vi "Periodic Tasks.vi"   [LabVIEW 2012]
doc: "This VI runs in parallel to other tasks. It can contain as many user-defined periodic loops as you need. These can carry out PID or other sorts of timed response."
uses:
  <vilib>/Rock Robotics/SystemInterfaces/Utilities/FPGA_UtilitiesLED Source.ctl
  <vilib>/Rock Robotics/SystemInterfaces/Utilities/FPGA_UtilitiesLED State.ctl
  Robot Global Data.vi
types:
  T1 = cluster{"Case":dbl, "VisionTrack":bool, "ShootEnableWheels":bool, "Shoot":bool, "ManualExtend":dbl, "ManualRotate":dbl, "YCoord":dbl, "FlipUp":bool, "RotDeadband":dbl, "ExtDeadband":dbl, "ExtPOT":dbl, "RotPOT":dbl, "WheelFSpd":dbl, "WheelBSpd":dbl, "ServoPositions":cluster{"FlipperLeftUp":dbl, "FlipperLeftDown":dbl, "FlipperRightUp":dbl, "FlipperRightDown":dbl, "KickerLeftBack":dbl, "KickerLeftForward":dbl, "KickerRightBack":dbl, "KickerRightForward":dbl}, "POTPositions":cluster{"Setpoint 1":dbl, "Setpoint 2":dbl, "Setpoint 3":dbl, "Setpoint 4":dbl, "RotLow":dbl, "RotHigh":dbl, "ExtLow":dbl, "ExtHigh":dbl}, "ClimberHooked":bool}
  T2 = typedef "WPI_DigitalInputDevRef.ctl" = cluster{"DevStatus":errorcluster, "DIO Channel":T3, "Digital Module":T4}
  T3 = typedef "FPGA_DIOChannel.ctl" = enum8{"DIO 1", "DIO 2", "DIO 3", "DIO 4", "DIO 5", "DIO 6", "DIO 7", "DIO 8", "DIO 9", "DIO 10", "DIO 11", "DIO 12", "DIO 13", "DIO 14", "Invalid"}
  T4 = typedef "FPGA_TypedefDigitalModule.ctl" = enum16{"Digital Module 1", "Digital Module 2"}
  T5 = cluster{"FlipperLeftUp":dbl, "FlipperLeftDown":dbl, "FlipperRightUp":dbl, "FlipperRightDown":dbl, "KickerLeftBack":dbl, "KickerLeftForward":dbl, "KickerRightBack":dbl, "KickerRightForward":dbl}
  T6 = cluster{"Setpoint 1":dbl, "Setpoint 2":dbl, "Setpoint 3":dbl, "Setpoint 4":dbl, "RotLow":dbl, "RotHigh":dbl, "ExtLow":dbl, "ExtHigh":dbl}
  T7 = typedef "WPI_AnalogChannelDevRef.ctl" = cluster{"DevStatus":errorcluster, "Analog Module":T8, "Analog Channel":T9}
  T8 = typedef "FPGA_TypedefAnalogModule.ctl" = enum16{"Analog Module 1", "Analog Module 2"}
  T9 = typedef "FPGA_AIChannel.ctl" = enum8{"AI 1", "AI 2", "AI 3", "AI 4", "AI 5", "AI 6", "AI 7", "AI 8", "Invalid"}
  T10 = typedef "WPI_RelayValue.ctl" = enum16{"Off", "On", "Forward", "Reverse"}
  T11 = cluster{"Case":dbl, "Extension":dbl, "Rotation":dbl, "WheelF":dbl, "WheelB":dbl, "Left Kicker":dbl, "Right Kicker":dbl, "Left Flipper":dbl, "Right Flipper":dbl, "Lights":T10}
  T12 = typedef "WPI_GyroDevRef.ctl" = cluster{"DevStatus":errorcluster, "Analog Module":T8, "Analog Channel":T9, "Offset":dbl, "Gain (VoltsPerDegree/Second)":dbl}
  T13 = typedef "WPI_EncoderDevRef.ctl" = cluster{"DevStatus":errorcluster, "EncoderIndex":T14, "CounterIndex":T15, "DistancePerCount":dbl, "Decoding Type":T16}
  T14 = typedef "FPGA_EncoderIdx.ctl" = enum8{"Enc 0", "Enc 1", "Enc 2", "Enc 3", "Invalid"}
  T15 = typedef "FPGA_CounterCtrSystemIndex.ctl" = enum8{"Ctr 0", "Ctr 1", "Ctr 2", "Ctr 3", "Ctr 4", "Ctr 5", "Ctr 6", "Ctr 7", "Invalid"}
  T16 = typedef "WPI_EncoderType.ctl" = enum16{"1x", "2x", "4x"}
  T17 = typedef "FPGA_UtilitiesLED State.ctl" = enum16{"Off", "On", "Toggle"}
  T18 = typedef "FPGA_UtilitiesLED Source.ctl" = enum16{"User LED", "FPGA LED"}
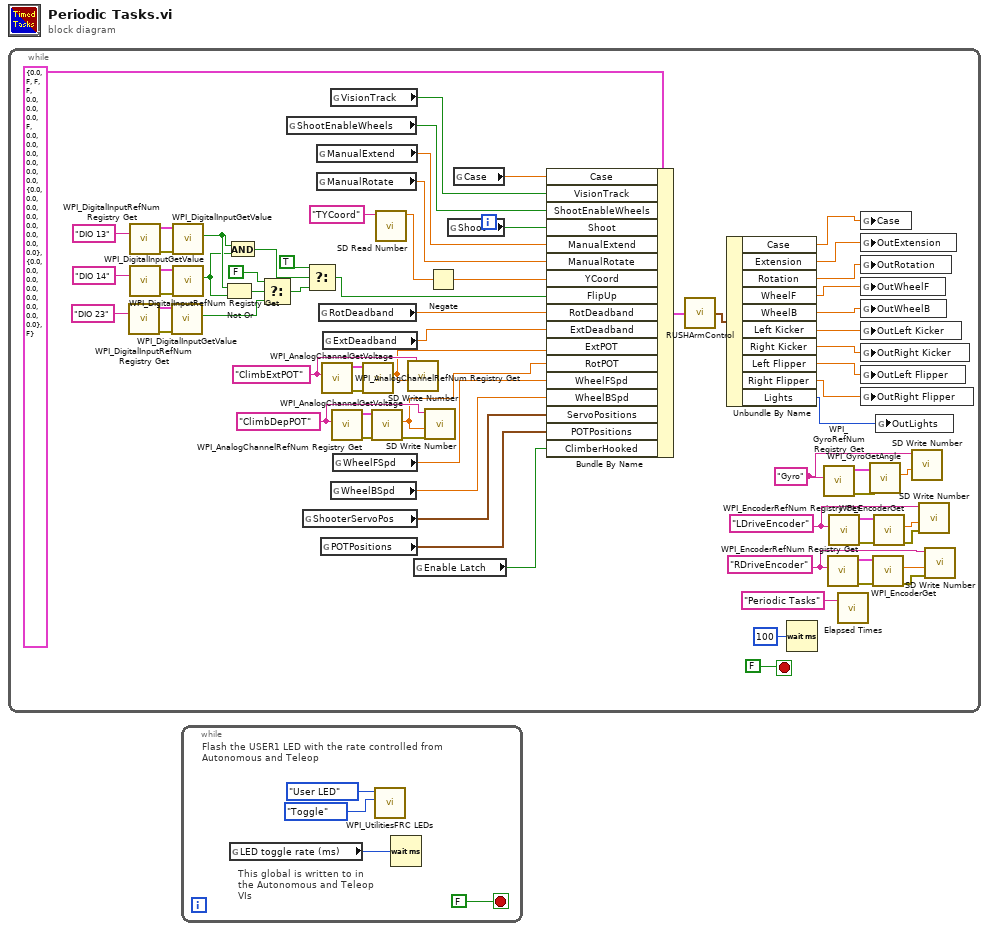
[diagram p0: block diagram]
diagram:
  n1 = while {
    stop <- FALSE stop-if-true
    w2 = "ClimbExtPOT" ("refnum name")
    w35 = "RDriveEncoder" ("refnum name")
    w31 = "LDriveEncoder" ("refnum name")
    w5 = "ClimbDepPOT" ("refnum name")
    w29 = "Gyro" ("refnum name")
    n2 = call <vilib>:"WPI_DigitalInputRefNum Registry Get.vi"("refnum name"="DIO 23") -> ("error out"=w11:errorcluster, "DigitalInputDevRef"=w8:T2)  [unwired: 9 in]
    n3 = call <vilib>:"WPI_DigitalInputRefNum Registry Get.vi"("refnum name"="DIO 13") -> ("error out"=w27:errorcluster, "DigitalInputDevRef"=w26:T2)  [unwired: 9 in]
    n4 = call <vilib>:"WPI_DigitalInputRefNum Registry Get.vi"("refnum name"="DIO 14") -> ("error out"=w20:errorcluster, "DigitalInputDevRef"=w21:T2)  [unwired: 9 in]
    n5 = call <vilib>:"WPI_DigitalInputGetValue.vi"("error in (no error)"=w11, "DigitalInputDevRef"=w8) -> ("Value"=w9:bool)  [unwired: 7 in, 2 out]
    n6 = call <vilib>:"WPI_DigitalInputGetValue.vi"("error in (no error)"=w27, "DigitalInputDevRef"=w26) -> ("Value"=w17:bool)  [unwired: 7 in, 2 out]
    n7 = call <vilib>:"WPI_DigitalInputGetValue.vi"("error in (no error)"=w20, "DigitalInputDevRef"=w21) -> ("Value"=w16:bool)  [unwired: 7 in, 2 out]
    n8 = Not Or(1:w16, 2:w17) -> (0:w15:bool)
    n9 = And(x=w17, y=w16) -> (x .and. y?=w19:bool)
    n10 = Select(t=FALSE, s=w15, f=w9) -> (s? t:f=w13:bool)
    n11 = global read "Robot Global Data.vi" "ShootEnableWheels"() -> (w55:bool)
    n12 = global read "Robot Global Data.vi" "ShooterServoPos"() -> (w47:T5)
    n13 = Select(t=TRUE, s=w19, f=w13) -> (s? t:f=w12:bool)
    n14 = global read "Robot Global Data.vi" "ManualExtend"() -> (w53:dbl)
    n15 = global read "Robot Global Data.vi" "ManualRotate"() -> (w52:dbl)
    n16 = global read "Robot Global Data.vi" "RotDeadband"() -> (w51:dbl)
    n17 = global read "Robot Global Data.vi" "POTPositions"() -> (w46:T6)
    n18 = call <vilib>:"WPI_AnalogChannelRefNum Registry Get.vi"("refnum name"=w2) -> ("error out"=w68:errorcluster, "AIDeviceRef"=w3:T7)  [unwired: 9 in]
    n19 = global read "Robot Global Data.vi" "ExtDeadband"() -> (w50:dbl)
    n20 = global read "Robot Global Data.vi" "VisionTrack"() -> (w56:bool)
    n21 = global read "Robot Global Data.vi" "WheelBSpd"() -> (w48:dbl)
    n22 = call <vilib>:"WPI_AnalogChannelRefNum Registry Get.vi"("refnum name"=w5) -> ("error out"=w63:errorcluster, "AIDeviceRef"=w62:T7)  [unwired: 9 in]
    n23 = global read "Robot Global Data.vi" "WheelFSpd"() -> (w49:dbl)
    n24 = call <vilib>:"WPI_AnalogChannelGetVoltage.vi"("error in (no error)"=w68, "AIDeviceRef"=w3) -> ("Voltage"=w1:dbl)  [unwired: 7 in, 2 out]
    n25 = call <vilib>:"WPI_AnalogChannelGetVoltage.vi"("error in (no error)"=w63, "AIDeviceRef"=w62) -> ("error out"=w6:errorcluster, "Voltage"=w4:dbl)  [unwired: 7 in, 1 out]
    n26 = call <vilib>:"SD Read Number.vi"("Name"="TYCoord") -> ("Numeric"=w24:dbl)  [unwired: 8 in, 2 out]
    n27 = call <vilib>:"SD Write Number.vi"("Numeric"=w1, "Name"=w2) -> ()  [unwired: 8 in, 2 out]
    n28 = global read "Robot Global Data.vi" "Enable Latch"() -> (w7:bool)
    n29 = call <vilib>:"SD Write Number.vi"("error in"=w6, "Numeric"=w4, "Name"=w5) -> ()  [unwired: 7 in, 2 out]
    n30 = Negate(x=w24) -> (-x=w23:dbl)
    n31 = global read "Robot Global Data.vi" "Shoot"() -> (w54:bool)
    n32 = global read "Robot Global Data.vi" "Case"() -> (w57:dbl)
    n33 = Bundle By Name(cluster=T1 {"Case"=0.0, "VisionTrack"=FALSE, "ShootEnableWheels"=FALSE, "Shoot"=FALSE, "ManualExtend"=0.0, "ManualRotate"=0.0, "YCoord"=0.0, "FlipUp"=FALSE, "RotDeadband"=0.0, "ExtDeadband"=0.0, "ExtPOT"=0.0, "RotPOT"=0.0, "WheelFSpd"=0.0, "WheelBSpd"=0.0, "ServoPositions"={"FlipperLeftUp"=0.0, "FlipperLeftDown"=0.0, "FlipperRightUp"=0.0, "FlipperRightDown"=0.0, "KickerLeftBack"=0.0, "KickerLeftForward"=0.0, "KickerRightBack"=0.0, "KickerRightForward"=0.0}, "POTPositions"={"Setpoint 1"=0.0, "Setpoint 2"=0.0, "Setpoint 3"=0.0, "Setpoint 4"=0.0, "RotLow"=0.0, "RotHigh"=0.0, "ExtLow"=0.0, "ExtHigh"=0.0}, "ClimberHooked"=FALSE} ("In Cluster"), "Case"=w57, "VisionTrack"=w56, "ShootEnableWheels"=w55, "Shoot"=w54, "ManualExtend"=w53, "ManualRotate"=w52, "YCoord"=w23, "FlipUp"=w12, "RotDeadband"=w51, "ExtDeadband"=w50, "ExtPOT"=w1, "RotPOT"=w4, "WheelFSpd"=w49, "WheelBSpd"=w48, "ServoPositions"=w47, "POTPositions"=w46, "ClimberHooked"=w7) -> (w59:T1)
    n34 = call "RUSHArmControl.vi"("In Cluster"=w59) -> ("Out Cluster"=w58:T11)
    n35 = Unbundle By Name(w58) -> ("Case"=w45:dbl, "Extension"=w44:dbl, "Rotation"=w43:dbl, "WheelF"=w42:dbl, "WheelB"=w41:dbl, "Left Kicker"=w40:dbl, "Right Kicker"=w39:dbl, "Left Flipper"=w38:dbl, "Right Flipper"=w37:dbl, "Lights"=w28:T10)
    n36 = Wait (ms)(milliseconds to wait=u32 100) -> ()  [unwired: 1 out]
    n37 = call <vilib>:"WPI_GyroRefNum Registry Get.vi"("refnum name"=w29) -> ("error out"=w69:errorcluster, "GyroDevRef"=w70:T12)  [unwired: 9 in]
    n38 = call <vilib>:"WPI_EncoderRefNum Registry Get.vi"("refnum name"=w35) -> ("error out"=w65:errorcluster, "EncoderDevRef"=w64:T13)  [unwired: 9 in]
    n39 = call <vilib>:"WPI_EncoderRefNum Registry Get.vi"("refnum name"=w31) -> ("error out"=w66:errorcluster, "EncoderDevRef"=w67:T13)  [unwired: 9 in]
    n40 = call "Elapsed Times.vi"("Call Name"="Periodic Tasks") -> ()  [unwired: 2 in, 1 out]
    n41 = global write "Robot Global Data.vi" "Case"(w45) -> ()
    n42 = global write "Robot Global Data.vi" "OutExtension"(w44) -> ()
    n43 = global write "Robot Global Data.vi" "OutRotation"(w43) -> ()
    n44 = global write "Robot Global Data.vi" "OutWheelF"(w42) -> ()
    n45 = global write "Robot Global Data.vi" "OutWheelB"(w41) -> ()
    n46 = global write "Robot Global Data.vi" "OutLeft Kicker"(w40) -> ()
    n47 = global write "Robot Global Data.vi" "OutRight Kicker"(w39) -> ()
    n48 = global write "Robot Global Data.vi" "OutLeft Flipper"(w38) -> ()
    n49 = global write "Robot Global Data.vi" "OutRight Flipper"(w37) -> ()
    n50 = call <vilib>:"WPI_GyroGetAngle.vi"("error in (no error)"=w69, "GyroDevRef"=w70) -> ("Angle"=w30:dbl)  [unwired: 6 in, 3 out]
    n51 = call <vilib>:"WPI_EncoderGet.vi"("error in (no error)"=w65, "EncoderDevRef"=w64) -> ("error out"=w32:errorcluster, "Distance"=w36:dbl)  [unwired: 4 in, 4 out]
    n52 = call <vilib>:"WPI_EncoderGet.vi"("error in (no error)"=w66, "EncoderDevRef"=w67) -> ("error out"=w34:errorcluster, "Distance"=w33:dbl)  [unwired: 4 in, 4 out]
    n53 = global write "Robot Global Data.vi" "OutLights"(w28) -> ()
    n54 = call <vilib>:"SD Write Number.vi"("Numeric"=w30, "Name"=w29) -> ()  [unwired: 8 in, 2 out]
    n55 = call <vilib>:"SD Write Number.vi"("error in"=w34, "Numeric"=w33, "Name"=w31) -> ()  [unwired: 7 in, 2 out]
    n56 = call <vilib>:"SD Write Number.vi"("error in"=w32, "Numeric"=w36, "Name"=w35) -> ()  [unwired: 7 in, 2 out]
  }
  n57 = while {
    stop <- FALSE stop-if-true
    # "This global is written to in the Autonomous and Teleop VIs"
    # "Flash the USER1 LED with the rate controlled from Autonomous and Teleop"
    n58 = global read "Robot Global Data.vi" "LED toggle rate (ms)"() -> (w74:u32)
    n59 = call <vilib>:"WPI_UtilitiesFRC LEDs.vi"("State"=FPGA_UtilitiesLED_State."Toggle", "LED Type"=FPGA_UtilitiesLED_Source."User LED") -> ()  [unwired: 1 in, 9 out]
    n60 = Wait (ms)(milliseconds to wait=w74) -> ()  [unwired: 1 out]
  }
